vi "Set Injected Value static.vi"(8 "error in (no error)":errorcluster, 10 "Value":T1, 11 "Value in":refnum<class "Abs_Extended Float.lvclass">) -> (0 "error out":errorcluster, 3 "Value out":refnum<class "Abs_Extended Float.lvclass">)   [LabVIEW 2021, in "Fault-Injection_EXT.lvclass"]
uses:
  Fault-Injection_EXT.lvclass
  Value Type.ctl
  <vilib>/TSA/Abstract Data Classes/Abs_Types/Extended Float/Abs_Extended Float.lvclass
  C:/Program Files (x86)/National Instruments/LabVIEW 2021/vi.lib/TSA/Abstract Data Classes/Abs_Types/Extended Float/Abs_Extended Float.lvclass
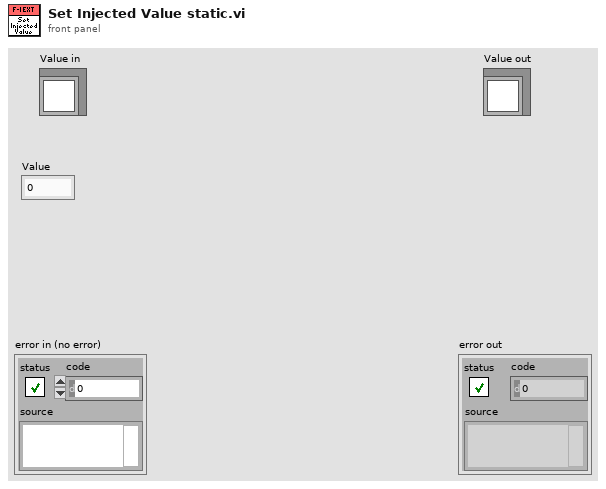
[diagram p1: front panel]
types:
  T1 = typedef "Fault-Injection_EXT.lvclass/Value Type.ctl" = ext
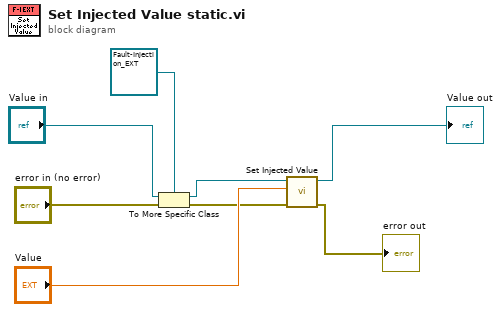
[diagram p0: block diagram]
diagram:
  n1 = To More Specific Class(target class=refnum<class "Fault-Injection_EXT.lvclass"> refnum ("Fault-Injection_EXT.lvclass"), reference="Value in", error in="error in (no error)") -> (specific class reference=w2:refnum<class "Fault-Injection_EXT.lvclass">, error out=w5:errorcluster)
  n2 = call-dynamic "Set Injected Value.vi"("error in (no error)"=w5, "Value"="Value", "Fault-Injection_Boolean in"=w2) -> ("error out"=→"error out":errorcluster, "Fault-Injection_Boolean out"=→"Value out":refnum<class "Fault-Injection_EXT.lvclass">)  [unwired: 7 in]
